vi "PH_Cont-601k_PowerUnit.contents.vi"   [LabVIEW 2014, in "PH_Cont-601k_PowerUnit.lvlib"]
doc: "This class is forseen to control a PreAmp Power Unit. Actually it controls several device layer classes. The head itself is fully operational, but should be used via the PHELIX_Sequencer class only. It has an own state machine.\n\nThis class is part of the PHELIX application layer."
uses:
  PH_Cont-601k_PowerUnit.lvlib
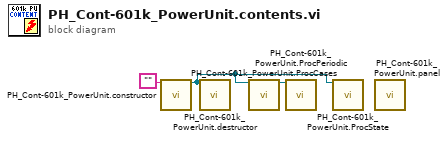
[diagram p0: block diagram]
diagram:
  n1 = call "PH_Cont-601k_PowerUnit.constructor.vi"("name"="") -> ("i ref out"=w1:refnum<vi>)  [unwired: 16 in, 2 out]
  n2 = call "PH_Cont-601k_PowerUnit.destructor.vi"("i ref in"=w1) -> ()  [unwired: 18 in, 1 out]
  n3 = call "PH_Cont-601k_PowerUnit.ProcCases.vi"("i ref in"=w1) -> ("i ref out"=w3:refnum<vi>)  [unwired: 16 in, 2 out]
  n4 = call "PH_Cont-601k_PowerUnit.ProcPeriodic.vi"("i ref in"=w3) -> ()  [unwired: 16 in, 3 out]
  n5 = call "PH_Cont-601k_PowerUnit.ProcState.vi"("i ref in"=w1) -> ()  [unwired: 16 in, 3 out]
  n6 = call "PH_Cont-601k_PowerUnit.panel.vi"() -> ()  [unwired: 1 in]
